vi "BLE characteristic to data.vi"(7 "ADC resolution":T1, 8 "Error In":errorcluster, 10 "characteristic value":u8[](array[numeric])) -> (0 "Error Out":errorcluster, 2 "Data value":sgl[](array[numeric]))   [LabVIEW 2016]
uses:
  Typedef/BLE - ADC Resolution.ctl
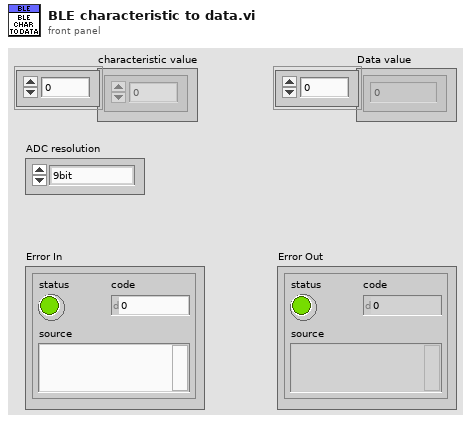
[diagram p1: front panel]
types:
  T1 = typedef "BLE - ADC Resolution.ctl" = enum16{"9bit", "10bit", "11bit", "12bit"}
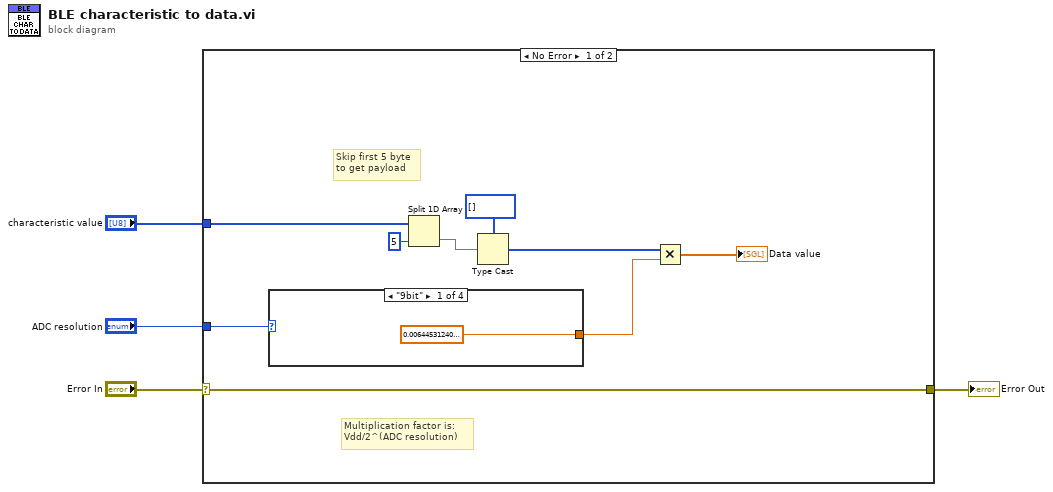
[diagram p0: block diagram]
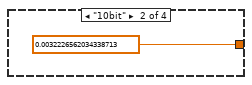
[diagram p2: hidden frame]
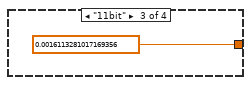
[diagram p3: hidden frame]
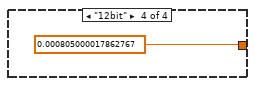
[diagram p4: hidden frame]
diagram:
  n1 = case shown="No Error" "Error In" {
    selector: "Error In" -> [w7 w18]
    tunnel: "characteristic value" -> [w8 _]
    tunnel: [w7 w18] -> w2
    tunnel: "ADC resolution" -> [w5 _]
    frame No Error {
      # "Multiplication factor is:\nVdd/2^(ADC resolution)"
      # "Skip first 5 byte \nto get payload"
      n2 = case shown="\"9bit\"" w5 {
        tunnel: [sgl 0.0064453124 sgl 0.0032226562 sgl 0.0016113281 sgl 0.000805] -> w12
        frame "9bit" {
        }
        frame "10bit" {
        }
        frame "11bit" {
        }
        frame "12bit" {
        }
      }
      n3 = Split 1D Array(array=w8, index=5) -> (second subarray=w11:u8[])  [unwired: 1 out]
      n4 = Type Cast(type=u16[] [], x=w11) -> (*(type *) &x=w9:u16[])
      n5 = Multiply(x=w9, y=w12) -> (x*y=→"Data value":sgl[])
    }
    frame Error {
    }
  }
  "Error Out" <- w2
